vi "PB_command_diss.vi"(9 "refocus_param":T2, 10 "commands":T3(array[cluster]), 11 "Refocus?":bool) -> (2 "PB_Commands":T1(array[cluster]), 3 "Exp_time":dbl[](array[numeric]), 5 "Number_repetitions":i32[](array[numeric]))   [LabVIEW 2018]
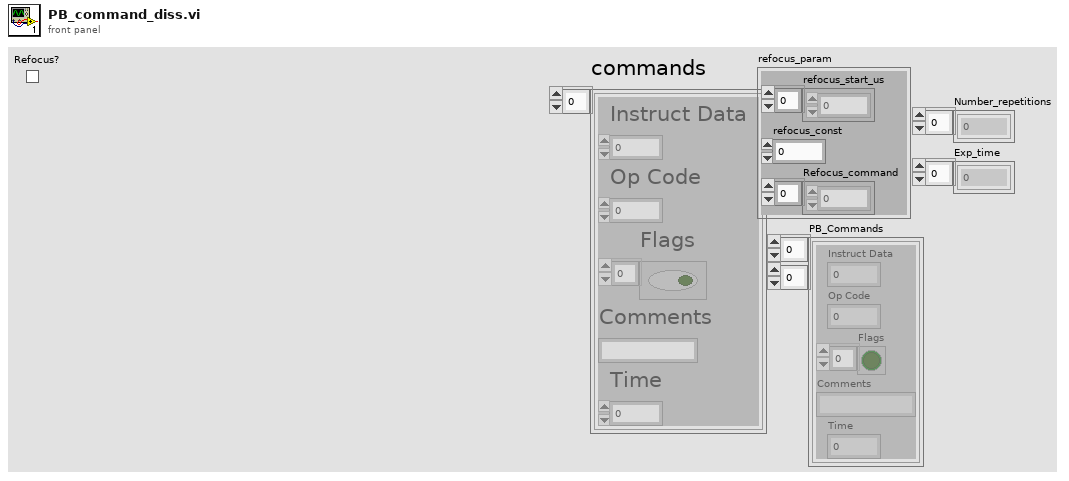
[diagram p1: front panel]
types:
  T1 = cluster{"Instruct Data":i32, "Op Code":i32, "Flags":bool[], "Comments":string, "Time":dbl}[][]
  T2 = cluster{"refocus_start_us":u32[], "refocus_const":dbl, "Refocus_command":dbl[]}
  T3 = cluster{"Instruct Data":i32, "Op Code":i32, "Flags":bool[], "Comments":string, "Time":dbl}[]
  T4 = cluster{"Instruct Data":i32, "Op Code":i32, "Flags":bool[], "Comments":string, "Time":dbl}
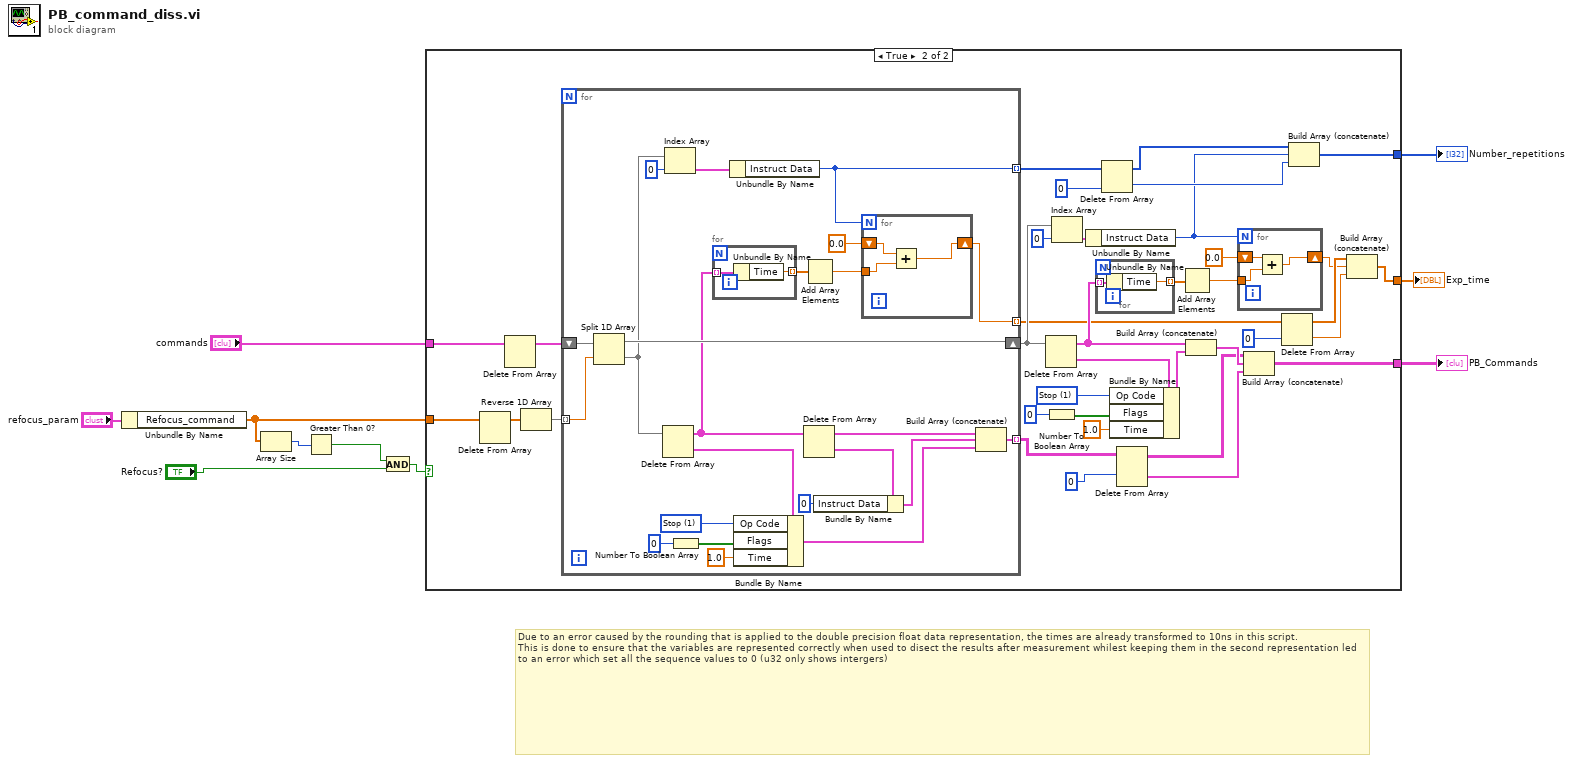
[diagram p0: block diagram]
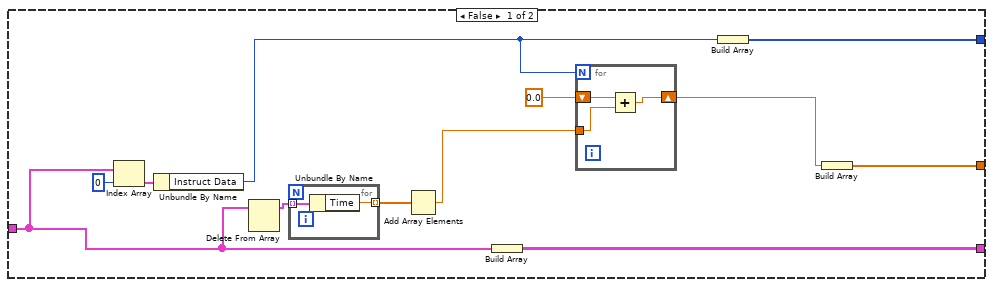
[diagram p2: hidden frame]
diagram:
  # "Due to an error caused by the rounding that is applied to the double precision float data representation, the times are already transformed to 10ns in this script. \nThis is done to ensure that the variables are represented correctly when used to disect the results after measurement whilest keeping them in the second representation led to an error which set all the sequence values to 0 (u32 only shows intergers)"
  n1 = Unbundle By Name("refocus_param") -> ("Refocus_command"=w5:dbl[])
  n2 = Array Size(array=w5) -> (size(s)=w4:i32)
  n3 = Greater Than 0?(x=w4) -> (x > 0?=w3:bool)
  n4 = And(x=w3, y="Refocus?") -> (x .and. y?=w7:bool)
  n5 = case shown="True" w7 {
    tunnel: "commands" -> [w19 w61]
    tunnel: [w22 w44] -> w9
    tunnel: w5 -> [_ w43]
    tunnel: [w11 w28] -> w1
    tunnel: [w16 w38] -> w2
    frame False {
      n6 = Index Array(array=w19, index=0) -> (element=w20:T4)
      n7 = Unbundle By Name(w20) -> ("Instruct Data"=w13:i32)
      n8 = Delete From Array(array=w19) -> (array with subset deleted=w18:T3)  [unwired: 2 in, 1 out]
      n9 = for {
        tunnel: w18 -> [w27] mode=indexing
        tunnel: [w26] -> w17 mode=indexing
        n10 = Unbundle By Name(w27) -> ("Time"=w26:dbl)
      }
      n11 = Add Array Elements(numeric array=w17) -> (sum=w15:dbl)
      n12 = Build Array(w19) -> (w22:T1)
      n13 = for {
        N: w13 -> [_]
        tunnel: w15 -> [w25]
        shift-right: [w23] -> w12
        shift-left: 0.0 -> [w24]
        n14 = Add(x=w24, y=w25) -> (x+y=w23:dbl)
      }
      n15 = Build Array(w13) -> (w16:i32[])
      n16 = Build Array(w12) -> (w11:dbl[])
    }
    frame True {
      w59 = 1 items=["Continue", "Stop", "Loop", "End Loop", "JSR", "RTS", "Branch", "Long Delay", "Wait"] ("Op Code 2")
      n17 = Delete From Array(array=w43) -> (array with subset deleted=w62:dbl[])  [unwired: 2 in, 1 out]
      n18 = Delete From Array(array=w61) -> (array with subset deleted=w60:T3)  [unwired: 2 in, 1 out]
      n19 = Reverse 1D Array(array=w62) -> (reversed array=w63:dbl[])
      n20 = for {
        shift-right: [w87] -> w52
        shift-left: w60 -> [w90]
        tunnel: w63 -> [w91] mode=indexing
        tunnel: [w83] -> w49 mode=indexing
        tunnel: [w71] -> w42 mode=indexing
        tunnel: [w69] -> w33 mode=indexing
        w88 = 1 items=["Continue", "Stop", "Loop", "End Loop", "JSR", "RTS", "Branch", "Long Delay", "Wait"] ("Op Code 2")
        n21 = Split 1D Array(array=w90, index=w91) -> (first subarray=w87:T3, second subarray=w75:T3)
        n22 = Delete From Array(array=w75) -> (deleted portion=w89:T4, array with subset deleted=w74:T3)  [unwired: 2 in]
        n23 = Index Array(array=w75, index=0) -> (element=w76:T4)
        n24 = Number To Boolean Array(number=0) -> (Boolean array=w84:bool[])
        n25 = for {
          tunnel: w74 -> [w96] mode=indexing
          tunnel: [w95] -> w73 mode=indexing
          n26 = Unbundle By Name(w96) -> ("Time"=w95:dbl)
        }
        n27 = Unbundle By Name(w76) -> ("Instruct Data"=w71:i32)
        n28 = Bundle By Name(cluster=w89, "Op Code"=w88, "Flags"=w84, "Time"=1.0) -> (w78:T4)
        n29 = Delete From Array(array=w74) -> (deleted portion=w82:T4, array with subset deleted=w80:T3)  [unwired: 2 in]
        n30 = Add Array Elements(numeric array=w73) -> (sum=w72:dbl)
        n31 = Bundle By Name(cluster=w82, "Instruct Data"=0) -> (w79:T4)
        n32 = for {
          N: w71 -> [_]
          tunnel: w72 -> [w93]
          shift-right: [w92] -> w69
          shift-left: 0.0 -> [w94]
          n33 = Add(x=w94, y=w93) -> (x+y=w92:dbl)
        }
        n34 = Build Array (concatenate)(w80, w79, w78) -> (w83:T3)
      }
      n35 = Delete From Array(array=w52) -> (deleted portion=w55:T4, array with subset deleted=w45:T3)  [unwired: 2 in]
      n36 = Number To Boolean Array(number=0) -> (Boolean array=w56:bool[])
      n37 = Index Array(array=w52, index=0) -> (element=w51:T4)
      n38 = Unbundle By Name(w51) -> ("Instruct Data"=w36:i32)
      n39 = for {
        tunnel: w45 -> [w68] mode=indexing
        tunnel: [w67] -> w37 mode=indexing
        n40 = Unbundle By Name(w68) -> ("Time"=w67:dbl)
      }
      n41 = Delete From Array(array=w42, index=0) -> (deleted portion=w39:i32, array with subset deleted=w40:i32[])  [unwired: 1 in]
      n42 = Bundle By Name(cluster=w55, "Op Code"=w59, "Flags"=w56, "Time"=1.0) -> (w54:T4)
      n43 = Delete From Array(array=w49, index (row)=0) -> (deleted portion=w47:T3, array with subset deleted=w48:T1)  [unwired: 2 in]
      n44 = Add Array Elements(numeric array=w37) -> (sum=w35:dbl)
      n45 = Build Array (concatenate)(w45, w54) -> (w50:T3)
      n46 = for {
        N: w36 -> [_]
        tunnel: w35 -> [w65]
        shift-right: [w64] -> w30
        shift-left: 0.0 -> [w66]
        n47 = Add(x=w66, y=w65) -> (x+y=w64:dbl)
      }
      n48 = Build Array (concatenate)(w48, w50, w47) -> (w44:T1)
      n49 = Delete From Array(array=w33, index=0) -> (deleted portion=w29:dbl, array with subset deleted=w31:dbl[])  [unwired: 1 in]
      n50 = Build Array (concatenate)(w40, w36, w39) -> (w38:i32[])
      n51 = Build Array (concatenate)(w31, w30, w29) -> (w28:dbl[])
    }
  }
  "PB_Commands" <- w9
  "Number_repetitions" <- w2
  "Exp_time" <- w1
